vi "Zero Phase Filter (obs, CDB).vi"(7 "init/cont (init:F)":bool, 9 "Forward Coefficients":dbl[](array[numeric]), 10 "Reverse Coefficients":dbl[](array[numeric]), 11 "X":cdb[](array[numeric])) -> (0 "error":i32, 3 "Filtered X":cdb[](array[numeric]))   [LabVIEW 2017, in "NI_AALBase.lvlib"]
doc: "Applies a zero phase filter to an input sequence <B>X</B>. Wire data to the <B>X</B> input to determine the polymorphic instance to use or manually select the instance."
uses:
  NI_AALBase.lvlib
panel:
  # "This VI is obsolete !!!\nYou should replace this VI in your diagram with the Zero Phase Filter VI.\n\nNOTE: If you have wired to the init input of this obsolete VI, please be\n            aware that the new Zero Phase Filter VI does not have such input.\n            Because of the non-causal property of zero phase filter, you should\n            use Zero Phase Filter VI in single-shot mode, not continuous mode."
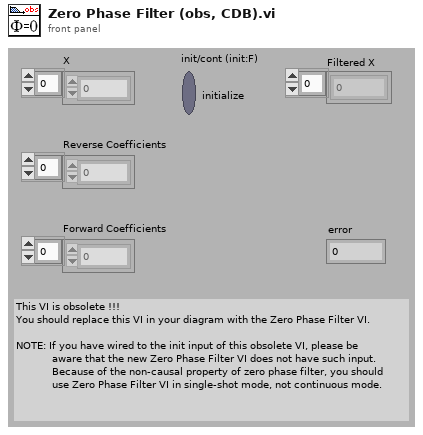
[diagram p1: front panel]
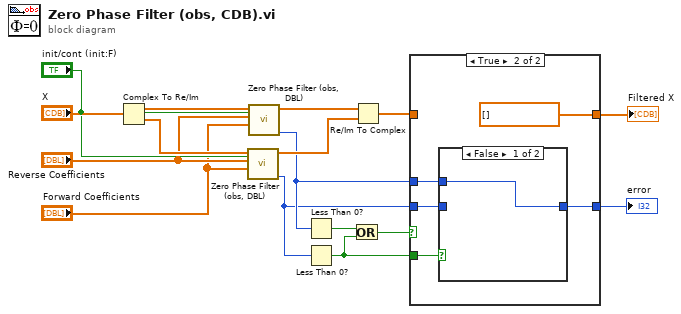
[diagram p0: block diagram]
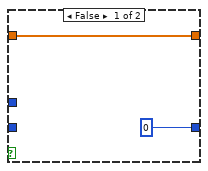
[diagram p2: hidden frame]
diagram:
  n1 = Complex To Re/Im(x + iy="X") -> (x=w15:dbl[], y=w14:dbl[])
  n2 = call "Zero Phase Filter (obs, DBL).vi"("init/cont (init:F)"="init/cont (init:F)", "Forward Coefficients"="Forward Coefficients", "Reverse Coefficients"="Reverse Coefficients", "X"=w14) -> ("error"=w7:i32, "Filtered X"=w11:dbl[])  [unwired: 6 in]
  n3 = call "Zero Phase Filter (obs, DBL).vi"("init/cont (init:F)"="init/cont (init:F)", "Forward Coefficients"="Forward Coefficients", "Reverse Coefficients"="Reverse Coefficients", "X"=w15) -> ("error"=w8:i32, "Filtered X"=w12:dbl[])  [unwired: 6 in]
  n4 = Less Than 0?(x=w8) -> (x < 0?=w13:bool)
  n5 = Less Than 0?(x=w7) -> (x < 0?=w4:bool)
  n6 = Or(x=w13, y=w4) -> (x .or. y?=w5:bool)
  n7 = Re/Im To Complex(1:w11, 2:w12) -> (0:w10:cdb[])
  n8 = case shown="True" w5 {
    tunnel: w10 -> [w18 _]
    tunnel: w4 -> [_ w23]
    tunnel: w7 -> [_ w22]
    tunnel: w8 -> [_ w21]
    tunnel: [0 ("error") w20] -> w6
    tunnel: [w18 cdb[] []] -> w9
    frame False {
    }
    frame True {
      n9 = case shown="False" w23 {
        tunnel: [w24 w25] -> w20
        tunnel: w22 -> [_ w25]
        tunnel: w21 -> [w24 _]
        frame False {
        }
        frame True {
        }
      }
    }
  }
  "Filtered X" <- w9
  "error" <- w6
